vi "CollectHardwareData.vi"(8 "Error In":errorcluster, 9 "ABLE Data Structures":T1, 10 "Hardware Data Structures":T2, 11 "Hardware Collect Data In":T3) -> (0 "Error Out":errorcluster, 3 "Hardware Collect Data Out":T3)   [LabVIEW 2012]
uses:
  HardwareCollectData.ctl
  PXI6229Data.ctl
  CurrentMeterData.ctl
  HardwareDataStructures.ctl
  HardwareLogData.ctl
  HardwareDisplayData.ctl
  ABLEDataStructures.ctl
  BPM.ctl
  ExperimentHardwareData.ctl
  ExperimentData.ctl
  AlarmData.ctl
  AlarmDatum.ctl
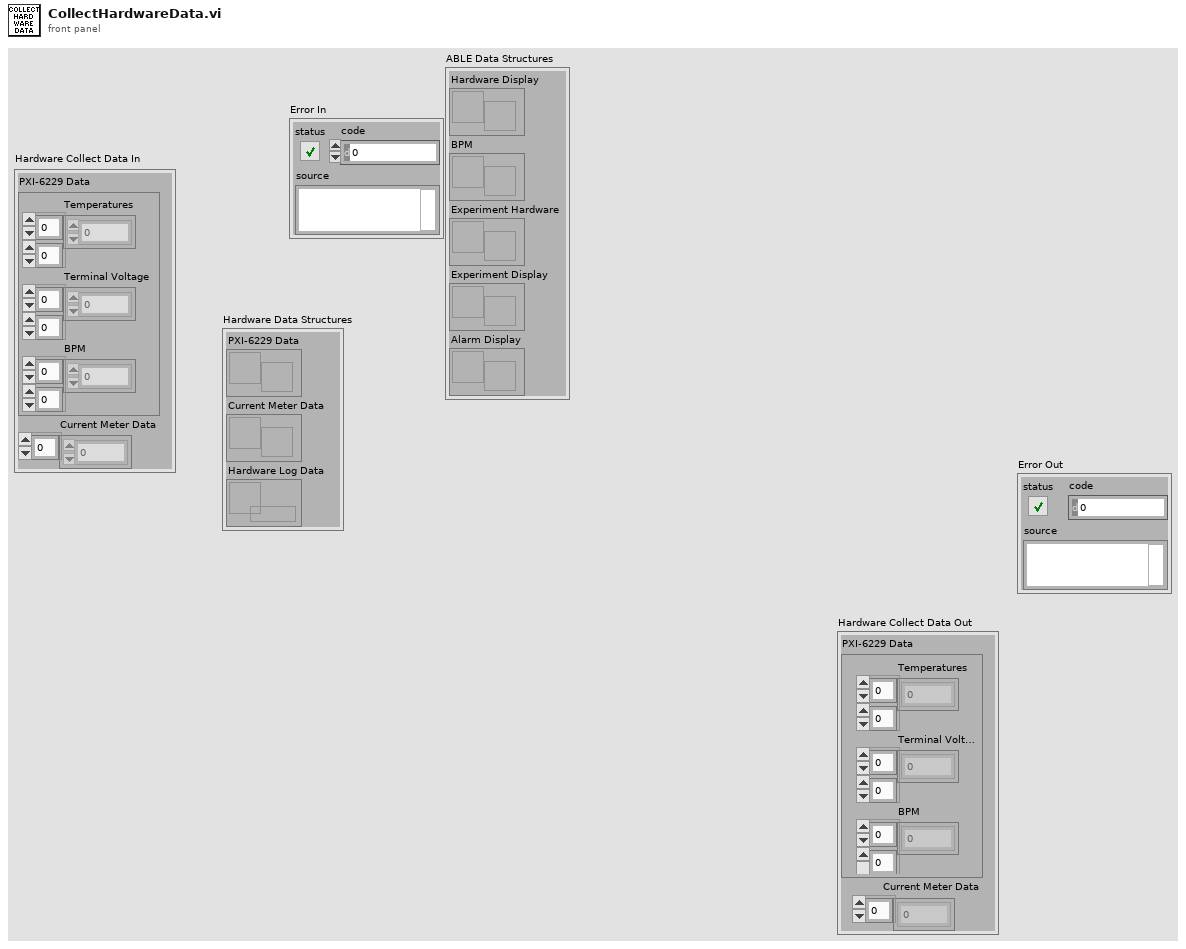
[diagram p1: front panel]
types:
  T1 = typedef "ABLEDataStructures.ctl" = cluster{"Hardware Display":refnum<notifier>, "BPM":refnum<notifier>, "Experiment Hardware":refnum<notifier>, "Experiment Display":refnum<notifier>, "Alarm Display":refnum<notifier>}
  T2 = typedef "HardwareDataStructures.ctl" = cluster{"PXI-6229 Data":refnum<notifier>, "Current Meter Data":refnum<notifier>, "Hardware Log Data":refnum<queue>}
  T3 = typedef "HardwareCollectData.ctl" = cluster{"PXI-6229 Data":T4, "Current Meter Data":T5}
  T4 = typedef "PXI6229Data.ctl" = cluster{"Temperatures":dbl[][], "Terminal Voltage":dbl[][], "BPM":dbl[][]}
  T5 = typedef "CurrentMeterData.ctl" = dbl[]
  T6 = typedef "HardwareDisplayData.ctl" = cluster{"Temperatures (C)":dbl[], "Terminal Voltage (MeV)":dbl, "Currents (A)":dbl[]}
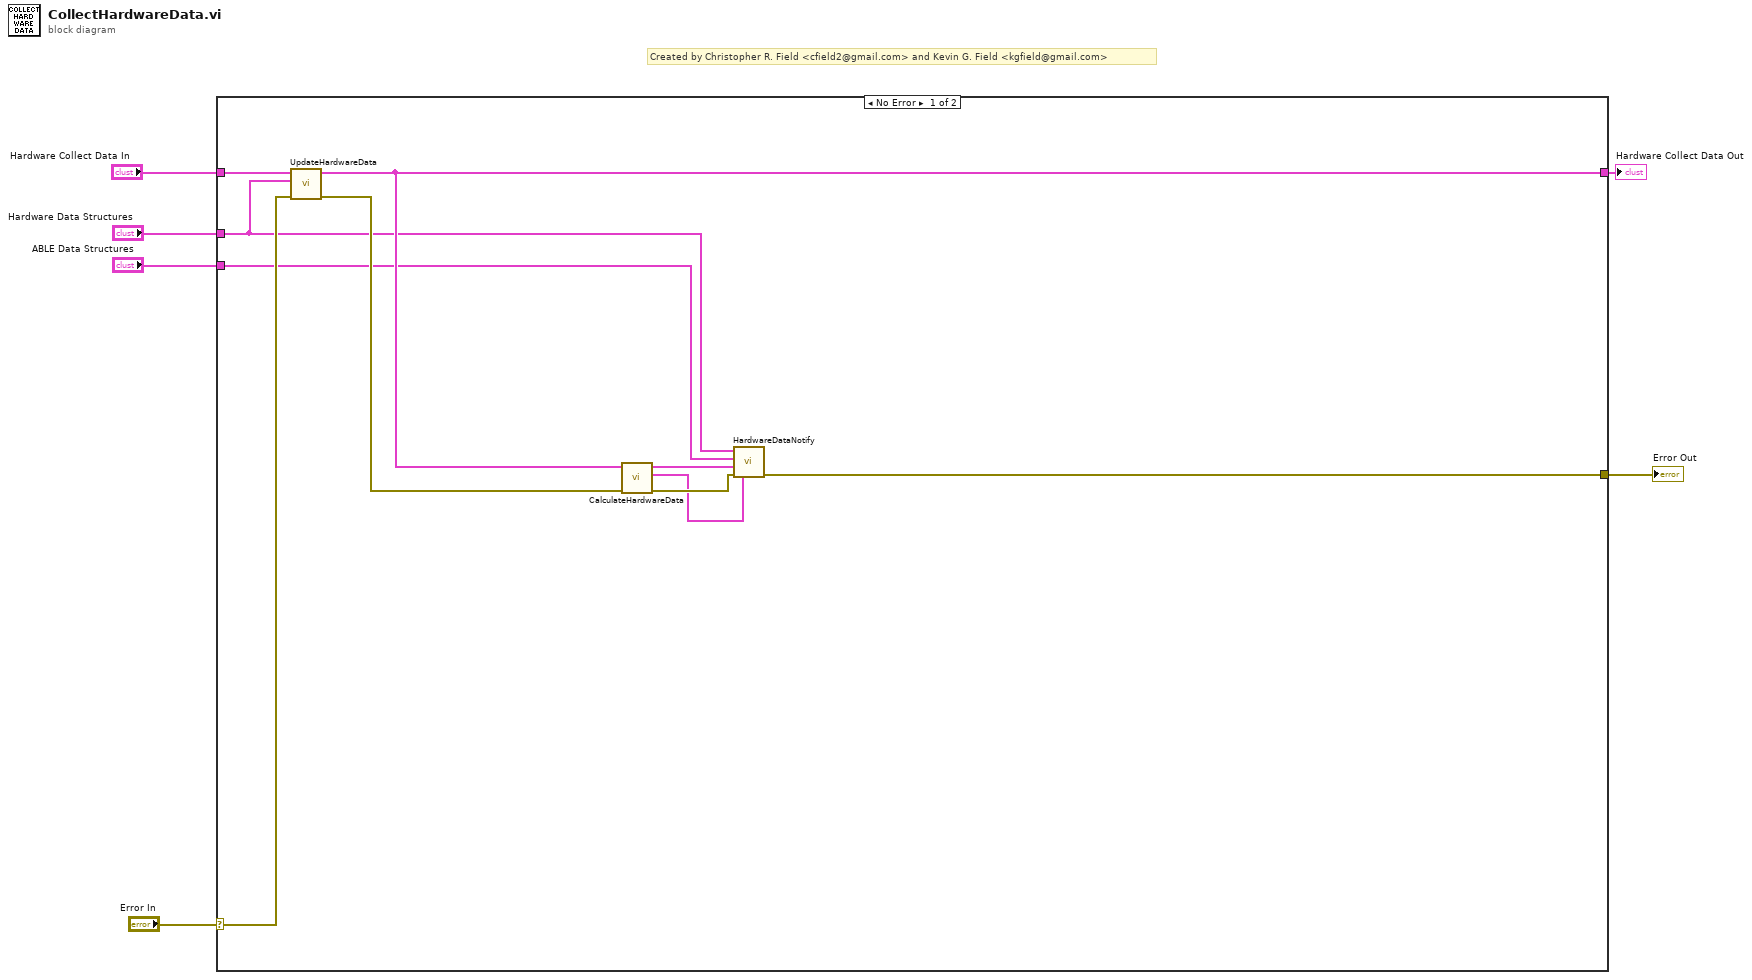
[diagram p0: block diagram]
diagram:
  # "Created by Christopher R. Field <cfield2@gmail.com> and Kevin G. Field <kgfield@gmail.com>"
  n1 = case shown="No Error" "Error In" {
    selector: "Error In" -> [w16 w18]
    tunnel: [w14 w18] -> w5
    tunnel: "Hardware Collect Data In" -> [w15 w17]
    tunnel: [w12 w17] -> w3
    tunnel: "Hardware Data Structures" -> [w8 _]
    tunnel: "ABLE Data Structures" -> [w9 _]
    frame No Error {
      n2 = call "UpdateHardwareData.vi"("Error In"=w16, "Hardware Data Structures"=w8, "Hardware Collect Data In"=w15) -> ("Error Out"=w13:errorcluster, "Hardware Collect Data Out"=w12:T3)  [unwired: 7 in]
      n3 = call "CalculateHardwareData.vi"("Error In"=w13, "Hardware Collect Data"=w12) -> ("Error Out"=w10:errorcluster, "BPM"=w7:cluster{dbl[], "Beam Profile":dbl[]}[], "Hardware Display Data"=w11:T6)  [unwired: 7 in]
      n4 = call "HardwareDataNotify.vi"("BPM"=w7, "Error In"=w10, "Hardware Display Data"=w11, "ABLE Data Structures"=w9, "Hardware Data Structures"=w8) -> ("Error Out"=w14:errorcluster)  [unwired: 6 in]
    }
    frame Error {
    }
  }
  "Error Out" <- w5
  "Hardware Collect Data Out" <- w3
